vi "transition to state.vi"(6 "timeout":i32, 8 "error in":errorcluster, 9 "state":T1, 10 "cmd fifo":refnum<k33>, 11 "notifier":refnum<notifier>) -> (0 "error out":errorcluster)   [LabVIEW 2013, in "Standard Engine Runtime.lvclass"]
uses:
  Standard Engine Runtime.lvclass
  engine state.ctl
  main engine/main engine.lvlib
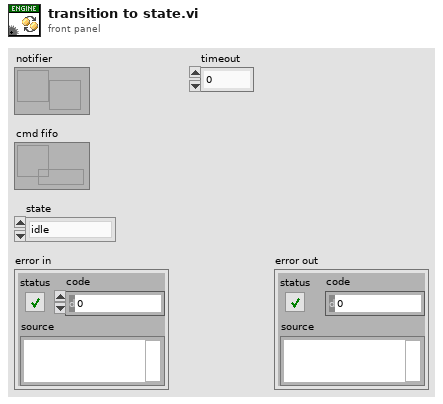
[diagram p1: front panel]
types:
  T1 = typedef "main engine.lvlib/engine state.ctl" = enum16{"idle", "configured", "running", "safe state", "exit"}
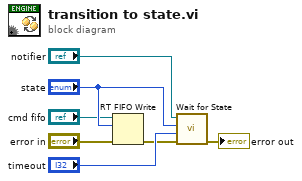
[diagram p0: block diagram]
diagram:
  n1 = RT FIFO Write(0:"cmd fifo", 1:"state", 3:"error in") -> (11:w3:errorcluster)  [unwired: 2 in, 3 out]
  n2 = call "Wait for State.vi"("error in"=w3, "timeout in ms"="timeout", "desired state"="state", "state notifier"="notifier") -> ("error out"=→"error out":errorcluster)  [unwired: 7 in]
